vi "Show error.vi"(8 "error in (no error)":errorcluster, 11 "DAQmxTaskContainer in":refnum<class "DAQmxTaskContainer.lvclass">) -> (0 "error out":errorcluster, 3 "DAQmxTaskContainer out":refnum<class "DAQmxTaskContainer.lvclass">)   [LabVIEW 2015, in "DAQmxTaskContainer.lvclass"]
uses:
  DAQmxTaskContainer.lvclass
  GeneralFunctionality/GeneralFunctionality.lvclass/GeneralFunctionality.ctl
  GeneralFunctionality/GeneralFunctionality.lvclass
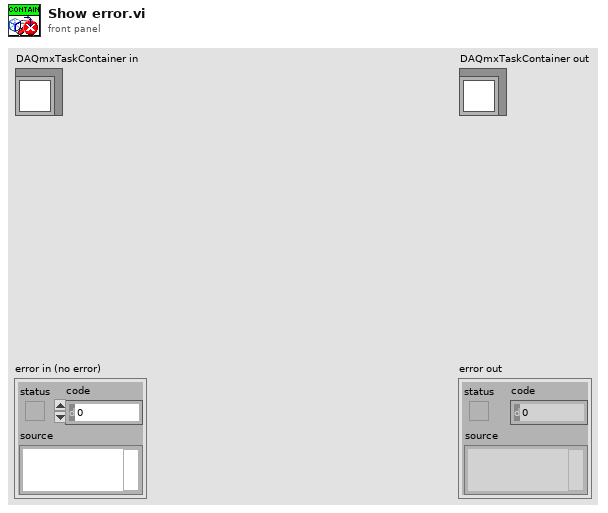
[diagram p1: front panel]
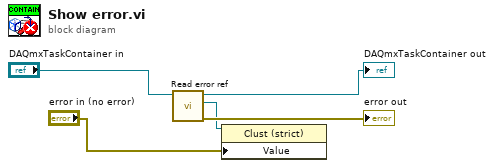
[diagram p0: block diagram]
diagram:
  n1 = call "Read error ref.vi"("GeneralFunctionality in"="DAQmxTaskContainer in") -> ("error out"=→"error out":errorcluster, "error"=w2:refnum<vi>, "GeneralFunctionality out"=→"DAQmxTaskContainer out":refnum<class "DAQmxTaskContainer.lvclass">)  [unwired: 8 in]
  n2 = property class="Clust (strict)"(reference=w2, "Value"="error in (no error)") -> ()  [unwired: 1 in, 2 out]
